vi "Coerce Waveform.vi"(1 "Lower Limit":dbl, 2 "Output Waveform":waveform(dbl), 3 "Upper Limit":dbl) -> (0 "Coerced Output Waveform":waveform(dbl))   [LabVIEW 2013]
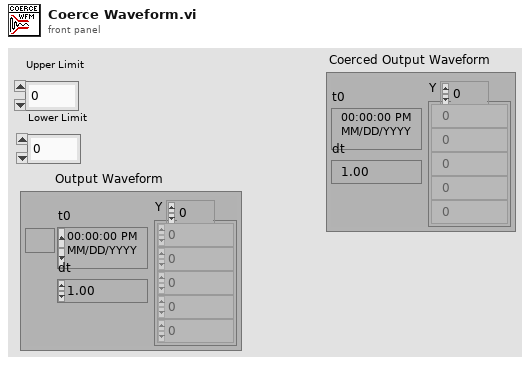
[diagram p1: front panel]
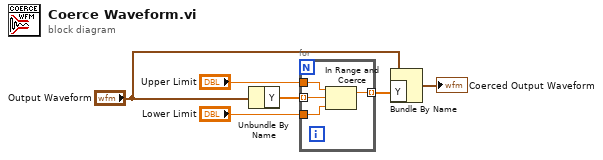
[diagram p0: block diagram]
diagram:
  n1 = Unbundle By Name("Output Waveform") -> ("Y"=w4:dbl[])
  n2 = for {
    tunnel: "Upper Limit" -> [w9]
    tunnel: "Lower Limit" -> [w8]
    tunnel: w4 -> [w10] mode=indexing
    tunnel: [w7] -> w3 mode=indexing
    n3 = In Range and Coerce(upper limit=w9, x=w10, lower limit=w8) -> (coerced(x)=w7:dbl)  [unwired: 1 out]
  }
  n4 = Bundle By Name(cluster="Output Waveform", "Y"=w3) -> (→"Coerced Output Waveform":waveform(dbl))
